vi "ExcelCreatModule.vi"() -> ()   [LabVIEW 2014]
uses:
  Data/Polymorphic VIs/Set Cell (String).vi
panel:
  in  "Count":cluster{"Sheet":i32, "Row":i32, "Column":i32}={"Sheet"=5, "Row"=129, "Column"=5}
  in  "Start Position 2":cluster{"Sheet":i32, "Row":i32, "Column":i32}
  in  "template (empty)":path=path "C:/Users/LENOVO/Desktop/CodeSpace GUI/data/SFP+ZR  Memory Map Module.xlsx" caption="模板（空）"
  in  "Start Position":cluster{"Sheet":i32, "Row":i32, "Column":i32}
  in  "File Name":path=path "C:/Users/LENOVO/Desktop/CodeSpace GUI/data/SFP+ZR  Memory Map Module1.xlsx"
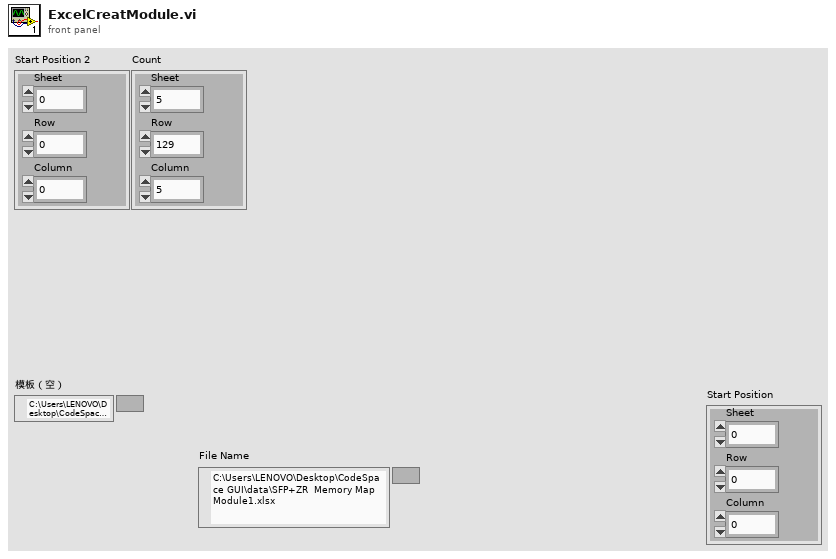
[diagram p1: front panel]
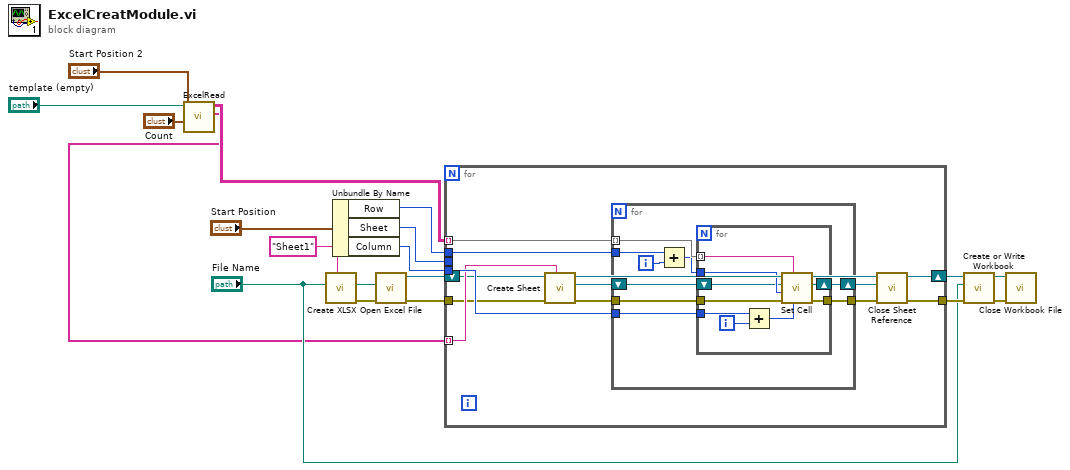
[diagram p0: block diagram]
diagram:
  n1 = call "ExcelRead.vi"("Count"="Count", "Start Position"="Start Position 2", "File Name"="template (empty)") -> ("Sheets Name"=w3:string[], "Values"=w4:string[][][])  [unwired: 7 in]
  n2 = call "Create XLSX.vi"("sheetname"="Sheet1", "File Name"="File Name") -> ("error out"=w10:errorcluster)  [unwired: 9 in]
  n3 = Unbundle By Name("Start Position") -> ("Row"=w17:i32, "Sheet"=w12:i32, "Column"=w11:i32)
  n4 = call "Open Excel File.vi"("error in (no error)"=w10, "File Name"="File Name") -> ("error out"=w9:errorcluster, "IWorkbook Reference Out"=w8:refnum<k24>)  [unwired: 8 in]
  n5 = for {
    tunnel: w4 -> [w30] mode=indexing
    tunnel: w12 -> [_]
    tunnel: w11 -> [w28]
    tunnel: w17 -> [w29]
    tunnel: w9 -> [w20]
    tunnel: [w25] -> w16
    shift-right: [w21] -> w15
    shift-left: w8 -> [w22]
    tunnel: w3 -> [w24] mode=indexing
    n6 = call "Create Sheet.vi"("Sheet Name (Sheet1)"=w24, "error in (no error)"=w20, "IWorkbook Reference"=w22) -> ("error out"=w19:errorcluster, "Sheet Reference"=w23:refnum<k24>, "IWorkbook Reference out"=w21:refnum<k24>)  [unwired: 6 in]
    n7 = for {
      tunnel: w30 -> [w39] mode=indexing
      tunnel: w29 -> [w37]
      tunnel: w28 -> [w36]
      tunnel: [w34] -> w26
      tunnel: w19 -> [w33]
      shift-right: [w32] -> w27
      shift-left: w23 -> [w31]
      i -> [w38]
      n8 = Add(x=w37, y=w38) -> (x+y=w35:i32)
      n9 = for {
        tunnel: w39 -> [w48] mode=indexing
        tunnel: w36 -> [w46]
        tunnel: w35 -> [w44]
        tunnel: [w42] -> w34
        tunnel: w33 -> [w41]
        shift-right: [w40] -> w32
        shift-left: w31 -> [w43]
        i -> [w47]
        n10 = Add(x=w46, y=w47) -> (x+y=w45:i32)
        n11 = call-poly "Set Cell.vi"("Column"=w45, "Value"=w48, "error in (no error)"=w41, "Row"=w44, "Sheet Reference"=w43) -> ("error out"=w42:errorcluster, "Sheet Reference out"=w40:refnum<k24>)  [unwired: 5 in]
      }
    }
    n12 = call "Close Sheet Reference.vi"("error in (no error)"=w26, "Sheet Reference"=w27) -> ("error out"=w25:errorcluster)  [unwired: 9 in]
  }
  n13 = call "Create or Write Workbook.vi"("error in (no error)"=w16, "File Name"="File Name", "IWorkbook Reference"=w15) -> ("error out"=w14:errorcluster, "IWorkbook Reference Out"=w13:refnum<k24>)  [unwired: 7 in]
  n14 = call "Close Workbook File.vi"("error in (no error)"=w14, "IWorkbook Reference"=w13) -> ()  [unwired: 9 in, 1 out]
